vi "Show Caller Items Dialog.vi"(9 "Theme":bool, 10 "Origin":string, 11 "Request VI Callers":refnum<vi>[](array[refnum])) -> ()   [LabVIEW 2019, in "Panther Dashboard.lvlib"]
uses:
  Panther Dashboard.lvlib
panel:
  in  "Results Listbox":i32(listbox)
  # "Note: Double Click an element to open it"
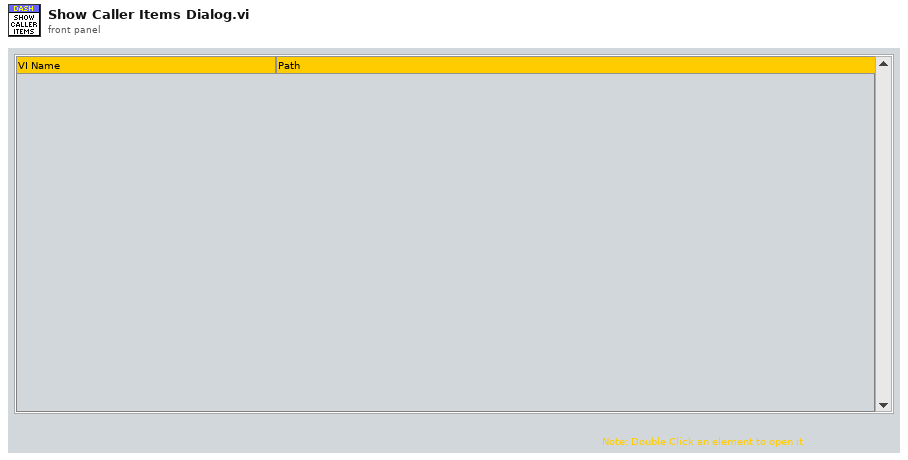
[diagram p1: front panel]
types:
  T1 = enum32{"Invalid", "Standard", "Closed", "Hidden", "Minimized", "Maximized"}
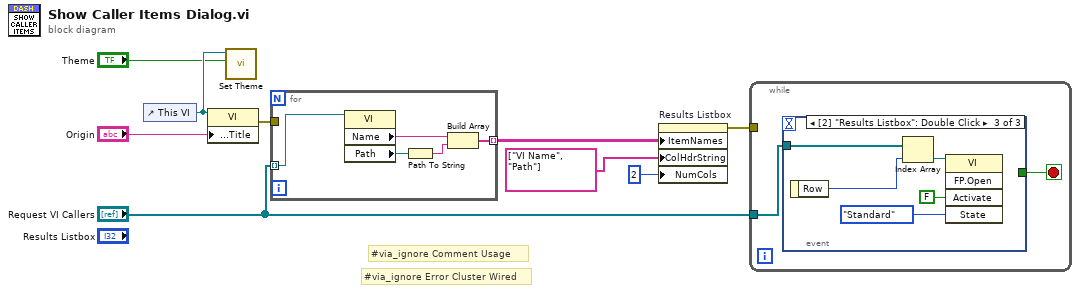
[diagram p0: block diagram]
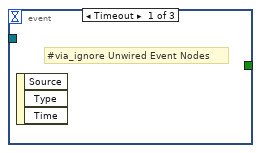
[diagram p2: hidden frame]
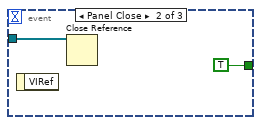
[diagram p3: hidden frame]
diagram:
  # "#via_ignore Error Cluster Wired"
  # "#via_ignore Comment Usage"
  n1 = control-ref of="This VI"() -> (w2:refnum<vi>)
  n2 = property class="VI"(reference=w2, "Front Panel.Title"="Origin") -> (error out=w8:errorcluster)  [unwired: 1 in, 1 out]
  n3 = call "Set Theme.vi"("Dark?"="Theme", "VI in"=w2) -> ()  [unwired: 10 in]
  n4 = for {
    tunnel: "Request VI Callers" -> [w14] mode=indexing
    tunnel: [w10] -> w5 mode=indexing
    tunnel: w8 -> [_]
    n5 = property class="VI"(reference=w14) -> ("Name"=w13:string, "Path"=w12:path)  [unwired: 1 in, 2 out]
    n6 = Path To String(path=w12) -> (string=w11:string)
    n7 = Build Array(w13, w11) -> (w10:string[])
  }
  n8 = property on="Results Listbox" class="MCListbox (strict)"("ItemNames"=w5, "ColHdrString"=string[] ["VI Name", "Path"] ("Column Header Strings[]"), "NumCols"=u32 2 ("Number of Columns")) -> (error out=w9:errorcluster)  [unwired: 2 in, 1 out]
  n9 = while {
    tunnel: "Request VI Callers" -> [w16]
    tunnel: w9 -> [_]
    stop <- w15 stop-if-true
    n10 = event shown="[2] \"Results Listbox\": Double Click" {
      selector: _ -> [_ _ _]
      dyn-events: _ -> [_ _ _]
      timeout: _ -> [_ _ _]
      tunnel: w16 -> [_ w18 w23]
      tunnel: [_ TRUE _] -> w15
      event Timeout {
        # "#via_ignore Unwired Event Nodes"
        n11 = event-data() -> ()  [unwired: 1 in, 3 out]
      }
      event Panel Close {
        n12 = event-data() -> ()  [unwired: 1 in, 1 out]
        n13 = Close Reference(reference=w18) -> ()  [unwired: 1 in, 1 out]
      }
      event "Results Listbox": Double Click {
        n14 = event-data() -> ("Row"=w22:i32)  [unwired: 1 in]
        n15 = Index Array(array=w23, index=w22) -> (element=w21:refnum<vi>)
        n16 = invoke class="VI" method="FP.Open"(reference=w21, "Activate"=FALSE ("Activate?"), "State"=T1."Standard") -> ()  [unwired: 2 in, 5 out]
      }
    }
  }
